vi "IO Enable.vi"(10 "enable":u8, 11 "channel":u8) -> ()   [LabVIEW 2021, in "vmmso.lvlib"]
doc: "DLL_API void WINAPI IOEnable(unsigned char channel, unsigned char enable);"
uses:
  vmmso.lvlib
  vmmso.dll
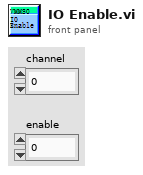
[diagram p1: front panel]
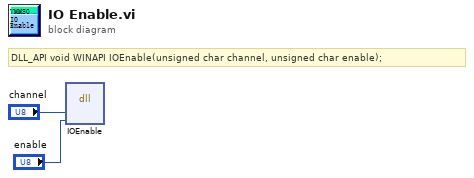
[diagram p0: block diagram]
diagram:
  # "DLL_API void WINAPI IOEnable(unsigned char channel, unsigned char enable);"
  n1 = dll-call lib="D:/labviewdemo/LabviewDemo 21/vmmso/vmmso.*" fn="IOEnable"("channel"="channel", "enable"="enable") -> ()  [unwired: 6 in, 2 out]
